vi "Select Data).vi"() -> ()   [LabVIEW 2024]
uses:
  <vilib>/addons/database/Connection.llb/Conn ObjectReference.ctl
  <vilib>/addons/database/NI_Database_API.lvlib
panel:
  in  "Boolean":bool
  out "resulting string":string
  in  "input 1":string
  out "error out":errorcluster
  out "connection reference 2":T1
  in  "error in (no error)":errorcluster
  in  "connection reference":T1
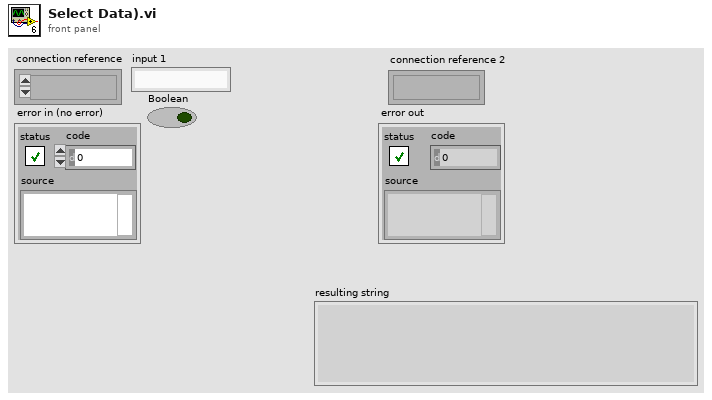
[diagram p1: front panel]
types:
  T1 = typedef "NI_Database_API.lvlib/Conn ObjectReference.ctl" = refnum<k1>
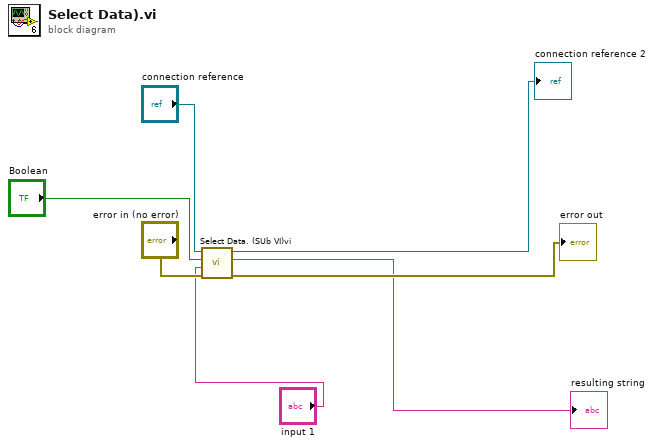
[diagram p0: block diagram]
diagram:
  n1 = call "Select Data. (SUb VI)vi.vi"("error in (no error)"="error in (no error)", "input 1"="input 1", "Boolean"="Boolean", "Refnum in"="connection reference") -> ("error out"=→"error out":errorcluster, "resulting string"=→"resulting string":string, "Refnum out"=→"connection reference 2":T1)  [unwired: 5 in]
